vi "DownsampleStage2_5160.vi"(8 "valid in":bool, 9 "reset":bool, 11 "Element":fxp<+/-,16,14>[](array[numeric])=[0.0, 0.0, 0.0, 0.0, 0.0, 0.0, 0.0, 0.0]) -> (0 "valid out":bool, 2 "Element 2":u64, 3 "Element 1":u64)   [LabVIEW 2013]
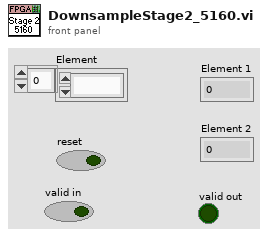
[diagram p1: front panel]
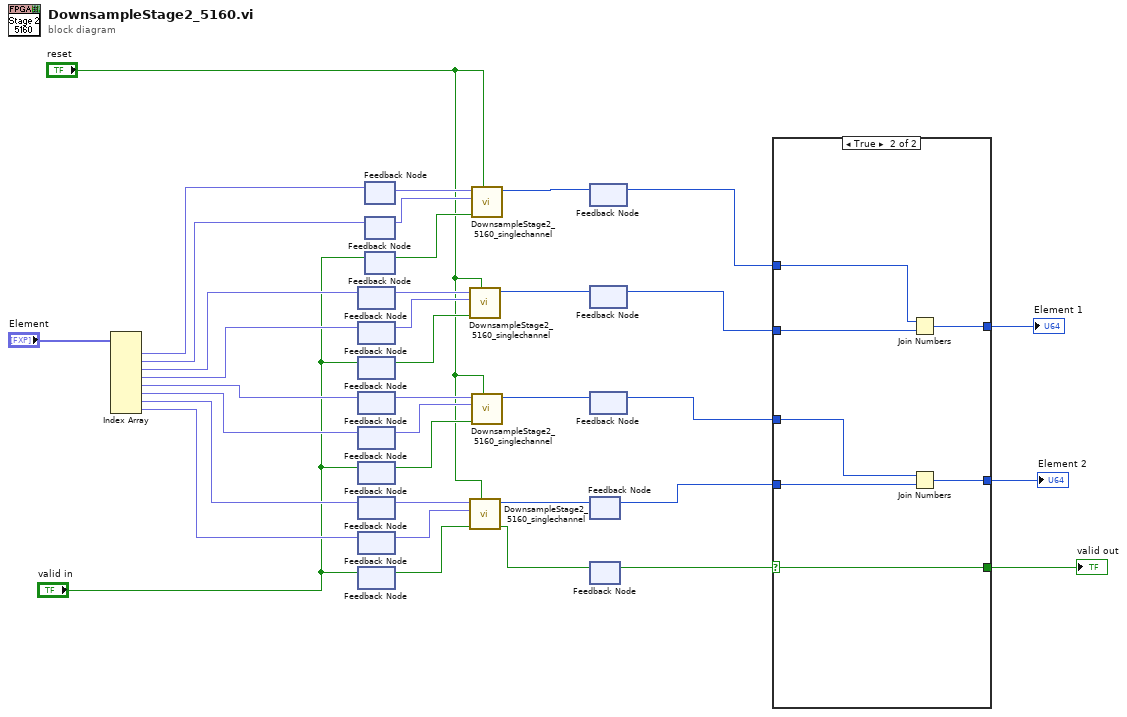
[diagram p0: block diagram]
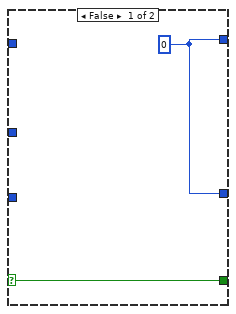
[diagram p2: hidden frame]
diagram:
  n1 = Index Array(array="Element") -> (element #1=w32:fxp<+/-,16,14>, element #2=w30:fxp<+/-,16,14>, element #3=w26:fxp<+/-,16,14>, element #4=w25:fxp<+/-,16,14>, element #5=w24:fxp<+/-,16,14>, element #6=w23:fxp<+/-,16,14>, element #7=w22:fxp<+/-,16,14>, element #8=w21:fxp<+/-,16,14>)  [unwired: 8 in]
  n2 = feedback #1() -> (w27:fxp<+/-,16,14>)  [unwired: 1 in]
  n3 = feedback-in #1(w26) -> ()
  n4 = feedback #2() -> (w19:fxp<+/-,16,14>)  [unwired: 1 in]
  n5 = feedback-in #2(w25) -> ()
  n6 = feedback #3() -> (w18:bool)  [unwired: 1 in]
  n7 = feedback-in #3("valid in") -> ()
  n8 = feedback #4() -> (w17:fxp<+/-,16,14>)  [unwired: 1 in]
  n9 = feedback-in #4(w24) -> ()
  n10 = feedback #5() -> (w15:fxp<+/-,16,14>)  [unwired: 1 in]
  n11 = feedback-in #5(w23) -> ()
  n12 = feedback #6() -> (w14:bool)  [unwired: 1 in]
  n13 = feedback-in #6("valid in") -> ()
  n14 = feedback #7() -> (w16:fxp<+/-,16,14>)  [unwired: 1 in]
  n15 = feedback-in #7(w22) -> ()
  n16 = feedback #8() -> (w13:fxp<+/-,16,14>)  [unwired: 1 in]
  n17 = feedback-in #8(w21) -> ()
  n18 = feedback #9() -> (w12:bool)  [unwired: 1 in]
  n19 = feedback-in #9("valid in") -> ()
  n20 = feedback #10() -> (w31:fxp<+/-,16,14>)  [unwired: 1 in]
  n21 = feedback-in #10(w32) -> ()
  n22 = feedback #11() -> (w29:fxp<+/-,16,14>)  [unwired: 1 in]
  n23 = feedback-in #11(w30) -> ()
  n24 = feedback #12() -> (w28:bool)  [unwired: 1 in]
  n25 = feedback-in #12("valid in") -> ()
  n26 = call "DownsampleStage2_5160_singlechannel.vi"("reset"="reset", "valid in"=w18, "I in"=w19, "Q in"=w27) -> ("IQ out"=w6:u32)  [unwired: 6 in, 1 out]
  n27 = call "DownsampleStage2_5160_singlechannel.vi"("reset"="reset", "valid in"=w12, "I in"=w13, "Q in"=w16) -> ("valid out"=w9:bool, "IQ out"=w10:u32)  [unwired: 6 in]
  n28 = call "DownsampleStage2_5160_singlechannel.vi"("reset"="reset", "valid in"=w28, "I in"=w29, "Q in"=w31) -> ("IQ out"=w11:u32)  [unwired: 6 in, 1 out]
  n29 = call "DownsampleStage2_5160_singlechannel.vi"("reset"="reset", "valid in"=w14, "I in"=w15, "Q in"=w17) -> ("IQ out"=w7:u32)  [unwired: 6 in, 1 out]
  n30 = feedback #13() -> (w4:u32)  [unwired: 1 in]
  n31 = feedback-in #13(w11) -> ()
  n32 = feedback #14() -> (w3:u32)  [unwired: 1 in]
  n33 = feedback-in #14(w6) -> ()
  n34 = feedback #15() -> (w2:u32)  [unwired: 1 in]
  n35 = feedback-in #15(w7) -> ()
  n36 = feedback #16() -> (w1:u32)  [unwired: 1 in]
  n37 = feedback-in #16(w10) -> ()
  n38 = feedback #17() -> (w8:bool)  [unwired: 1 in]
  n39 = feedback-in #17(w9) -> ()
  n40 = case shown="True" w8 {
    selector: w8 -> [w38 w44]
    tunnel: w4 -> [_ w42]
    tunnel: w3 -> [_ w41]
    tunnel: [w37 w45] -> w35
    tunnel: [w38 w44] -> w34
    tunnel: [w37 w43] -> w33
    tunnel: w2 -> [_ w40]
    tunnel: w1 -> [_ w39]
    frame False {
      w37 = u64 0
    }
    frame True {
      n41 = Join Numbers(hi=w42, lo=w41) -> ((hi.lo)=w45:u64)
      n42 = Join Numbers(hi=w40, lo=w39) -> ((hi.lo)=w43:u64)
    }
  }
  "Element 1" <- w35
  "valid out" <- w34
  "Element 2" <- w33
